vi "parse.vi"(8 "error in (no error)":errorcluster, 10 "DynamicFrameParser":refnum<class "DynamicFrameParser.lvclass">, 11 "MDILC in":refnum<class "MDILC.lvclass">) -> (0 "error out":errorcluster, 2 "ParseSuccessful":bool, 3 "MDILC out":refnum<class "MDILC.lvclass">)   [LabVIEW 2016, in "RTMDILC.lvlib" / "MDILC.lvclass"]
uses:
  MDILC.lvclass
  Common_RT_Modbus/DynamicFrameParser/DynamicFrameParser.lvclass
  Common_RT_ILC/ILC/ILC.lvclass
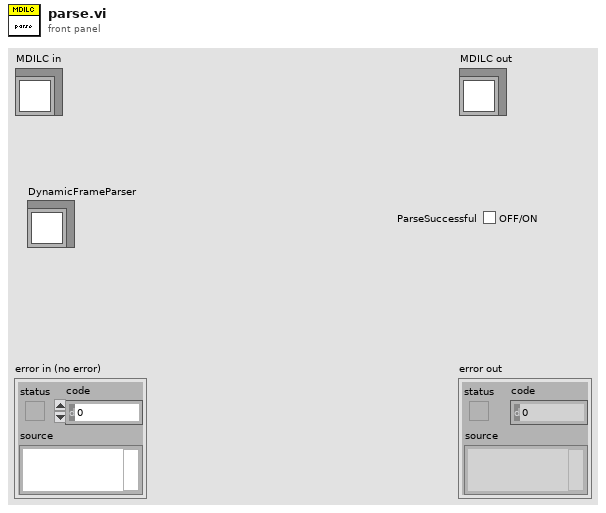
[diagram p1: front panel]
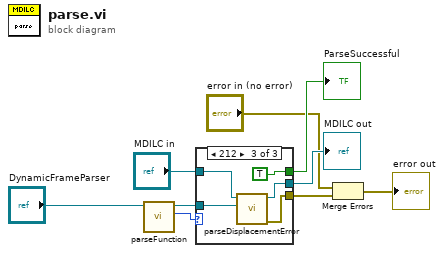
[diagram p0: block diagram]
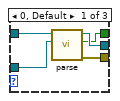
[diagram p2: hidden frame]
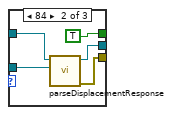
[diagram p3: hidden frame]
diagram:
  n1 = call "parseFunction.vi"("FrameParser in"="DynamicFrameParser") -> ("Function"=w8:u8, "FrameParser out"=w1:refnum<class "DynamicFrameParser.lvclass">)  [unwired: 8 in, 1 out]
  n2 = case shown="212" w8 {
    tunnel: "MDILC in" -> [w14 w19 w24]
    tunnel: [w13 w18 w23] -> w6
    tunnel: [w12 TRUE ("ParseSuccessful") TRUE ("ParseSuccessful")] -> w5
    tunnel: [w11 w16 w21] -> w4
    tunnel: w1 -> [w10 w15 w20]
    frame 0, Default {
      n3 = call-parent "parse.vi"("DynamicFrameParser"=w10, "ILC in"=w14) -> ("error out"=w11:errorcluster, "ParseSuccessful"=w12:bool, "ILC out"=w13:refnum<class "MDILC.lvclass">)  [unwired: 7 in]
    }
    frame 84 {
      n4 = call "parseDisplacementResponse.vi"("DynamicFrameParser"=w15, "MDILC in"=w19) -> ("error out"=w16:errorcluster, "MDILC out"=w18:refnum<class "MDILC.lvclass">)  [unwired: 8 in]
    }
    frame 212 {
      n5 = call "parseDisplacementError.vi"("DynamicFrameParser"=w20, "MDILC in"=w24) -> ("error out"=w21:errorcluster, "MDILC out"=w23:refnum<class "MDILC.lvclass">)  [unwired: 8 in]
    }
  }
  "MDILC out" <- w6
  "ParseSuccessful" <- w5
  n6 = Merge Errors("error in (no error)", w4) -> (→"error out":errorcluster)
